vi "test_MonoMoveAndGetSlitPositionInMM.vi"(0 "device selection":enum16{"monochromator", "CCD", "SCD"}(ring), 1 "Test should pass":bool=TRUE, 5 "set-up a connection":bool=TRUE, 9 "tear down connection":bool=TRUE, 11 "error in":errorcluster, 12 "Delay between send and receive [ms]":i32=100, 13 "wait for procedure to be finished [ms]":i32=4000) -> (10 "log-file path":path, 15 "error out":errorcluster)   [LabVIEW 2023]
uses:
  Classes/Mono/Monochromator.lvclass
  C:/Users/grju/Desktop/AbgelegteDokumente/Kunden/Horiba/horiba-labview-sdk/Source/Classes/GenericDevice/GenericDevice.lvclass
  <vilib>/addons/_JKI Toolkits/Caraya/classes/Assert/Assert Equal Value and Type_Variant.vi
  <vilib>/addons/_JKI Toolkits/Caraya/classes/Assert/Assert Not Error.vi
  <vilib>/addons/_JKI Toolkits/Caraya/classes/Test/Test.lvclass
  <vilib>/addons/_JKI Toolkits/Caraya/classes/Assert/Assert.lvclass
  <vilib>/Hampel Software Engineering/HSE Logger/hse-logger.lvlib
panel:
  # "Connector Pane"
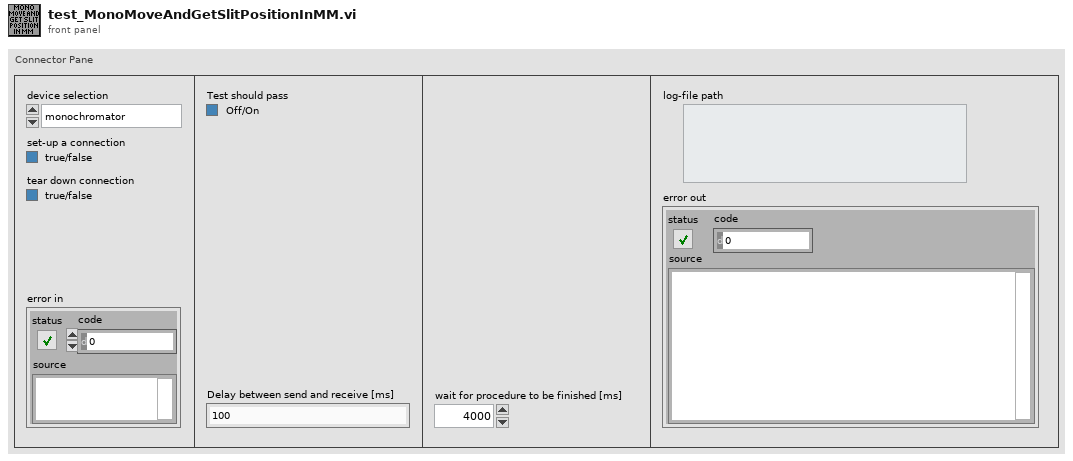
[diagram p1: front panel]
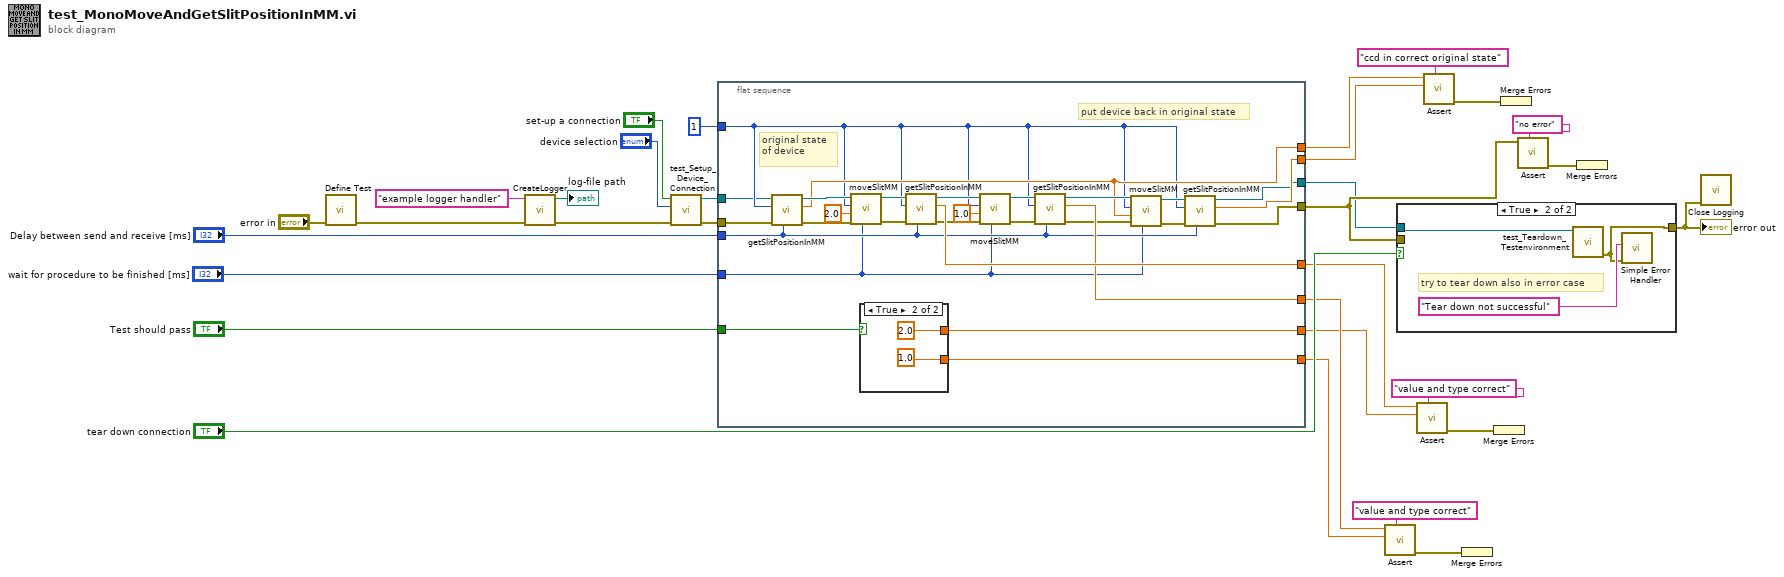
[diagram p0: block diagram]
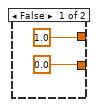
[diagram p2: hidden frame]
diagram:
  n1 = call <vilib>:"Define Test.vi"("error in (no error)"="error in") -> ("error out"=w4:errorcluster)  [unwired: 9 in, 1 out]
  n2 = call "CreateLogger.vi"("error in (no error)"=w4, "Handler Name"="example logger handler") -> ("error out"=w3:errorcluster, "log-file path"=→"log-file path":path)  [unwired: 8 in]
  n3 = call "test_Setup_Device_Connection.vi"("error in (no error)"=w3, "device selection"="device selection", "set-up a connection"="set-up a connection") -> ("error out"=w10:errorcluster, "Monochromator.lvclass"=w8:refnum<class "Monochromator.lvclass">)  [unwired: 5 in, 2 out]
  n4 = flat-sequence {
    tunnel: w10 -> [w33]
    tunnel: w8 -> [w32]
    tunnel: [w40] -> w22
    tunnel: "Test should pass" -> [w59]
    tunnel: [w41] -> w21
    tunnel: [w47] -> w20
    tunnel: [w58] -> w19
    tunnel: [w52] -> w18
    tunnel: [w57] -> w17
    tunnel: [w37] -> w14
    tunnel: [w42] -> w13
    tunnel: "Delay between send and receive [ms]" -> [w39]
    tunnel: "wait for procedure to be finished [ms]" -> [w38]
    tunnel: 1 ("type") -> [w35]
    frame #0 {
      # "put device back in original state"
      # "original state of device"
      n5 = call "getSlitPositionInMM.vi"("Delay between send and receive [ms]"=w39, "error in (no error)"=w33, "locationId"=w35, "Monochromator in"=w32) -> ("error out"=w55:errorcluster, "position"=w37:dbl, "Monochromator out"=w56:refnum<class "Monochromator.lvclass">)  [unwired: 5 in]
      n6 = call "moveSlitMM.vi"("Delay between send and receive [ms]"=w38, "error in (no error)"=w55, "position"=2.0, "locationId"=w35, "Monochromator in"=w56) -> ("error out"=w54:errorcluster, "Monochromator out"=w53:refnum<class "Monochromator.lvclass">)  [unwired: 3 in, 2 out]
      n7 = case shown="True" w59 {
        tunnel: [0.0 ("position") 1.0 ("position")] -> w58
        tunnel: [1.0 ("position") 2.0 ("position")] -> w57
        frame False {
        }
        frame True {
        }
      }
      n8 = call "getSlitPositionInMM.vi"("Delay between send and receive [ms]"=w39, "error in (no error)"=w54, "locationId"=w35, "Monochromator in"=w53) -> ("error out"=w48:errorcluster, "position"=w52:dbl, "Monochromator out"=w49:refnum<class "Monochromator.lvclass">)  [unwired: 5 in]
      n9 = call "moveSlitMM.vi"("Delay between send and receive [ms]"=w38, "error in (no error)"=w48, "position"=1.0, "locationId"=w35, "Monochromator in"=w49) -> ("error out"=w51:errorcluster, "Monochromator out"=w50:refnum<class "Monochromator.lvclass">)  [unwired: 3 in, 2 out]
      n10 = call "getSlitPositionInMM.vi"("Delay between send and receive [ms]"=w39, "error in (no error)"=w51, "locationId"=w35, "Monochromator in"=w50) -> ("error out"=w44:errorcluster, "position"=w47:dbl, "Monochromator out"=w45:refnum<class "Monochromator.lvclass">)  [unwired: 5 in]
      n11 = call "moveSlitMM.vi"("Delay between send and receive [ms]"=w38, "error in (no error)"=w44, "position"=w37, "locationId"=w35, "Monochromator in"=w45) -> ("error out"=w46:errorcluster, "Monochromator out"=w43:refnum<class "Monochromator.lvclass">)  [unwired: 3 in, 2 out]
      n12 = call "getSlitPositionInMM.vi"("Delay between send and receive [ms]"=w39, "error in (no error)"=w46, "locationId"=w35, "Monochromator in"=w43) -> ("error out"=w40:errorcluster, "position"=w42:dbl, "Monochromator out"=w41:refnum<class "Monochromator.lvclass">)  [unwired: 5 in]
    }
  }
  n13 = call-poly <vilib>:"Assert.vi"("Label"="value and type correct" ("Label (VI Title)"), "Y"=w19, "X"=w20) -> ("error out"=w30:errorcluster)  [unwired: 7 in, 1 out]
  n14 = case shown="True" "tear down connection" {
    tunnel: w21 -> [_ w66]
    tunnel: [w64 w65] -> w1
    tunnel: w22 -> [w64 _]
    frame False {
    }
    frame True {
      # "try to tear down also in error case"
      n15 = call "test_Teardown_Testenvironment.vi"("GenericDevice.lvclass"=w66) -> ("error out"=w65:errorcluster)  [unwired: 9 in, 1 out]
      n16 = call <vilib>:"Simple Error Handler.vi"("error source (\" \")"="Tear down not successful" ("error source (\" \")"), "error in (no error)"=w65) -> ()  [unwired: 3 in, 5 out]
    }
  }
  "error out" <- w1
  n17 = call-poly <vilib>:"Assert.vi"("Label"="value and type correct" ("Label (VI Title)"), "Y"=w17, "X"=w18) -> ("error out"=w29:errorcluster)  [unwired: 7 in, 1 out]
  n18 = call-poly <vilib>:"Assert.vi"("Label"="ccd in correct original state" ("Label (VI Title)"), "Y"=w13, "X"=w14) -> ("error out"=w16:errorcluster)  [unwired: 7 in, 1 out]
  n19 = Merge Errors(w30) -> ()  [unwired: 1 out]
  n20 = Merge Errors(w29) -> ()  [unwired: 1 out]
  n21 = Merge Errors(w16) -> ()  [unwired: 1 out]
  n22 = call-poly <vilib>:"Assert.vi"("Label"="no error" ("Label (VI Title)"), "Not Error?"=w22) -> ("error out"=w24:errorcluster)  [unwired: 8 in, 1 out]
  n23 = Merge Errors(w24) -> ()  [unwired: 1 out]
  n24 = call <vilib>:"Close Logging.vi"("error in"=w1) -> ()  [unwired: 10 in, 1 out]
